vi "XNET Database Get List.vi"(0 "IP address (localhost)":string, 11 "error in (no error)":errorcluster) -> (4 "array of alias":string[](array[string]), 6 "array of filepath":path[](array[path]), 15 "error out":errorcluster)   [LabVIEW 2018]
doc: "Gets the current list of databases on a system."
uses:
  nixlvapi.dll
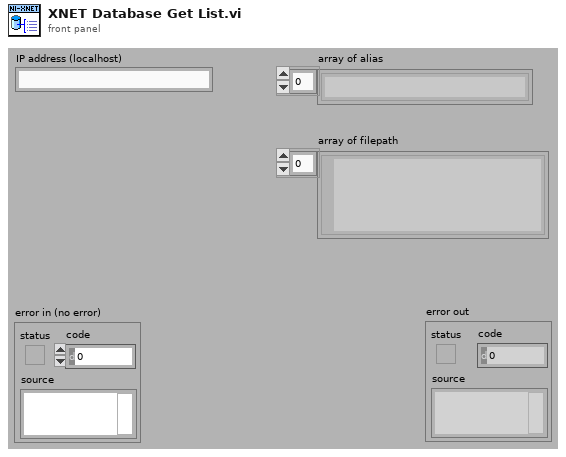
[diagram p1: front panel]
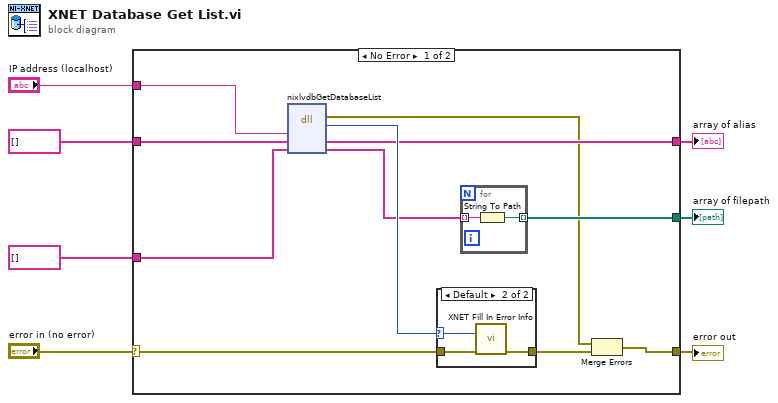
[diagram p0: block diagram]
diagram:
  n1 = case shown="No Error" "error in (no error)" {
    selector: "error in (no error)" -> [w17 w25]
    tunnel: [w9 w25] -> w7
    tunnel: "IP address (localhost)" -> [w15 _]
    tunnel: string[] [] ("array of alias") -> [w13 _]
    tunnel: [w14 _] -> w3
    tunnel: [w10 _] -> w2
    tunnel: string[] [] ("array of alias") -> [w12 _]
    frame No Error {
      n2 = dll-call lib="nixlvapi.*" fn="nixlvdbGetDatabaseList" ("nilvxaiu.dll:lvxenDatabaseDeleteObject")("IPAddress"=w15, "ArrayOfAlias"=w13, "ArrayOfFilepath"=w12) -> (error out=w8:errorcluster, "return type"=w16:i32, "ArrayOfAlias"=w14:string[], "ArrayOfFilepath"=w11:string[])  [unwired: 4 in, 1 out]
      n3 = case shown="Default" w16 {
        selector: w16 -> [_ w22]
        tunnel: w17 -> [w21 w23]
        tunnel: [w21 w24] -> w18
        frame 0 {
        }
        frame Default {
          n4 = call "XNET Fill In Error Info.vi"("status code"=w22, "error in"=w23) -> ("error out"=w24:errorcluster)  [unwired: 13 out]
        }
      }
      n5 = for {
        tunnel: w11 -> [w20] mode=indexing
        tunnel: [w19] -> w10 mode=indexing
        n6 = String To Path(string=w20) -> (path=w19:path)
      }
      n7 = Merge Errors(w8, w18) -> (w9:errorcluster)
    }
    frame Error {
    }
  }
  "error out" <- w7
  "array of filepath" <- w2
  "array of alias" <- w3
